vi "VI Server_MergeRefs.vi"(7 "VI Server Cluster 1":T1, 8 "error in":errorcluster, 11 "VI Server Cluster 2":T1) -> (0 "error out":errorcluster, 3 "VI Server Cluster Merged":T1)   [LabVIEW 2020, in "VI Server Toolkit LV2013.lvlib"]
doc: "Performs merging VI Server Clusters (two of them).\nUsage: access controls of dynamically/remote VI controls programmatically."
uses:
  VI Server Toolkit LV2013.lvlib
  VI Server_TypeDefs/VI Server_RefsCluster.ctl
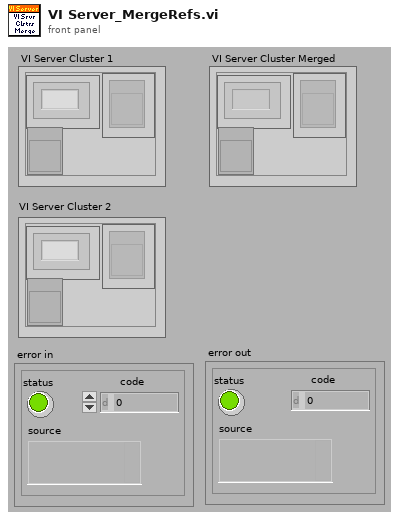
[diagram p1: front panel]
types:
  T1 = typedef "VI Server_RefsCluster.ctl" = cluster{"Labels":string[], "Refs":refnum<vi>[], "VI Ref":refnum<vi>}
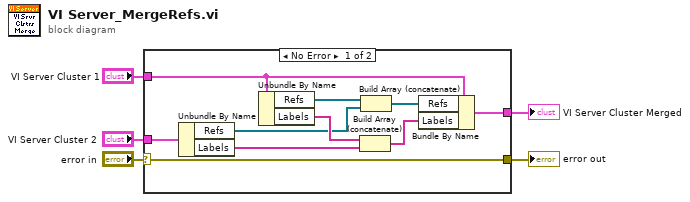
[diagram p0: block diagram]
diagram:
  n1 = case shown="No Error" "error in" {
    selector: "error in" -> [w10 w16]
    tunnel: "VI Server Cluster 2" -> [w8 _]
    tunnel: [w10 w16] -> w4
    tunnel: [w11 _] -> w2
    tunnel: "VI Server Cluster 1" -> [w9 _]
    frame No Error {
      n2 = Unbundle By Name(w8) -> ("Refs"=w6:refnum<vi>[], "Labels"=w7:string[])
      n3 = Unbundle By Name(w9) -> ("Refs"=w15:refnum<vi>[], "Labels"=w13:string[])
      n4 = Build Array (concatenate)(w13, w7) -> (w12:string[])
      n5 = Build Array (concatenate)(w15, w6) -> (w14:refnum<vi>[])
      n6 = Bundle By Name(cluster=w9, "Refs"=w14, "Labels"=w12) -> (w11:T1)
    }
    frame Error {
    }
  }
  "error out" <- w4
  "VI Server Cluster Merged" <- w2
